vi "Handle Mouse Down.vi"(8 "error in (no error)":errorcluster, 10 "Event Data":T2, 11 "Selector in":refnum<class "Selector.lvclass">) -> (0 "error out":errorcluster, 1 "Enable Change":bool, 3 "Selector out":refnum<class "Selector.lvclass">)   [LabVIEW 2019, in "Selector.lvclass"]
uses:
  Selector.lvclass
  <vilib>/Utility/miscctls.llb/LVPositionTypeDef.ctl
  Selector.lvclass/Selector.ctl
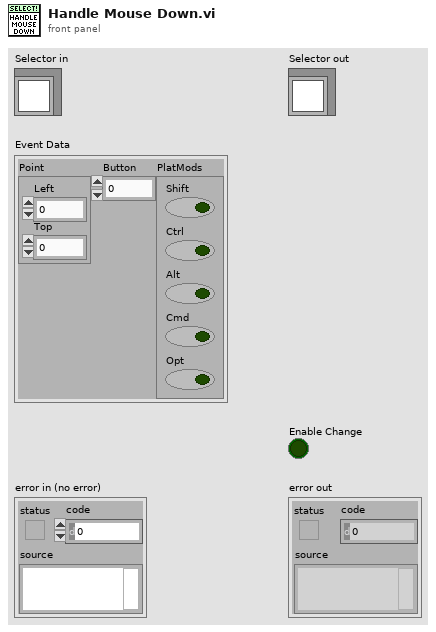
[diagram p1: front panel]
types:
  T1 = typedef "LVPositionTypeDef.ctl" = cluster{"Left":i32, "Top":i32}
  T2 = cluster{"Point":T1, "Button":u16, "PlatMods":cluster{"Shift":bool, "Ctrl":bool, "Alt":bool, "Cmd":bool, "Opt":bool}}
  T3 = typedef "LVRowAndColumnTypeDef.ctl" = cluster{"Row":i32, "Column":i32}
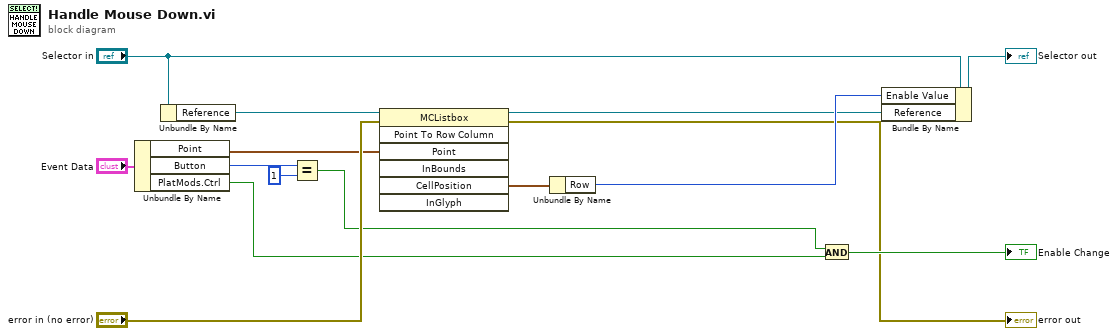
[diagram p0: block diagram]
diagram:
  n1 = Unbundle By Name("Event Data") -> ("Point"=w9:T1, "Button"=w8:u16, "PlatMods.Ctrl"=w6:bool)
  n2 = Unbundle By Name("Selector in") -> ("Reference"=w15:refnum<vi>)
  n3 = Equal?(x=w8, y=u16 1) -> (x = y?=w3:bool)
  n4 = invoke class="MCListbox" method="Point To Row Column"(reference=w15, error in="error in (no error)", "Point"=w9) -> (reference out=w1:refnum<vi>, error out=→"error out":errorcluster, "CellPosition"=w14:T3)  [unwired: 4 in, 4 out]
  n5 = Unbundle By Name(w14) -> ("Row"=w4:i32)
  n6 = And(x=w3, y=w6) -> (x .and. y?=→"Enable Change":bool)
  n7 = Bundle By Name(cluster="Selector in", "Enable Value"=w4, "Reference"=w1) -> (→"Selector out":refnum<class "Selector.lvclass">)
